vi "Write.vi"(8 "error in (no error)":errorcluster, 10 "Command To Write":string, 11 "VISA resource name":refnum<visa-resource-name>) -> (0 "error out":errorcluster, 3 "VISA resource name out":refnum<visa-resource-name>)   [LabVIEW 2018, in "EFD Ultimus V.lvlib"]
doc: "Writes a command to the Ultimus V unit, computes the checksum and sets the command to the correct format. For example, acceptable inputs are EK-- , UCccc, E8ccc. Refer to the Ultimus V manual for host format command formats."
uses:
  EFD Ultimus V.lvlib
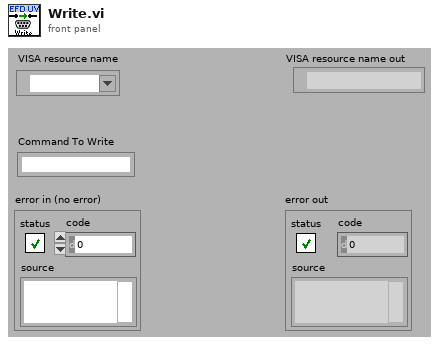
[diagram p1: front panel]
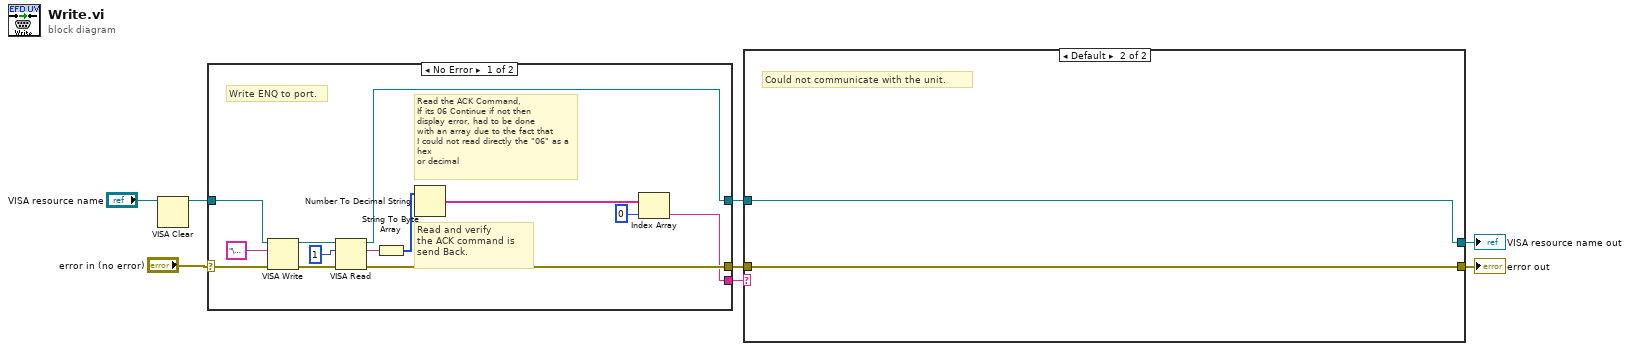
[diagram p0: block diagram]
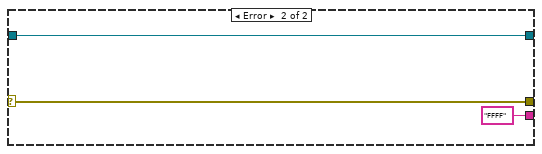
[diagram p2: hidden frame]
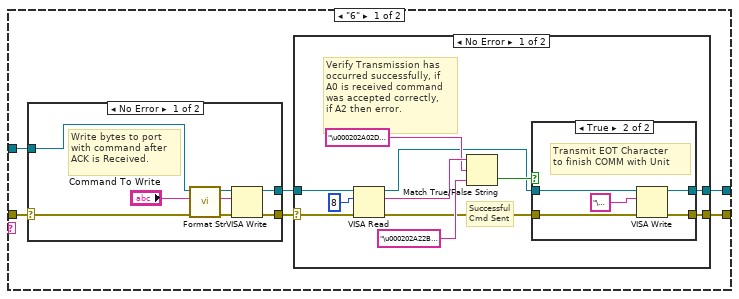
[diagram p3: hidden frame]
diagram:
  n1 = VISA Clear(VISA resource name="VISA resource name") -> (VISA resource name out=w4:refnum<visa-resource-name>)  [unwired: 1 in, 1 out]
  n2 = case shown="No Error" "error in (no error)" {
    selector: "error in (no error)" -> [w21 w24]
    tunnel: [w15 w23] -> w5
    tunnel: [w16 w24] -> w6
    tunnel: w4 -> [w20 w23]
    tunnel: [w10 "FFFF" ("read buffer")] -> w7
    frame No Error {
      # "Read the ACK Command,\nIf its 06 Continue if not then\ndisplay error, had to be done\nwith an array due to the fact that \nI could not read directly the \"06\" as a hex\nor decimal"
      # "Read and verify \nthe ACK command is \nsend Back."
      # "Write ENQ to port."
      n3 = VISA Write(VISA resource name=w20, write buffer="\u0005", error in (no error)=w21) -> (VISA resource name out=w18:refnum<visa-resource-name>, error out=w17:errorcluster)  [unwired: 1 out]
      n4 = VISA Read(VISA resource name=w18, byte count=u32 1, error in (no error)=w17) -> (VISA resource name out=w15:refnum<visa-resource-name>, read buffer=w14:string, error out=w16:errorcluster)  [unwired: 1 out]
      n5 = String To Byte Array(string=w14) -> (unsigned byte array=w13:u8[])
      n6 = Number To Decimal String(number=w13) -> (decimal integer string=w12:string[])  [unwired: 1 out]
      n7 = Index Array(array=w12, index=0) -> (element=w10:string)
    }
    frame Error {
    }
  }
  n8 = case shown="Default" w7 {
    tunnel: [w26 w62] -> w8
    tunnel: w5 -> [w28 w62]
    tunnel: w6 -> [w27 w61]
    tunnel: [w25 w61] -> w1
    frame "6" {
      n9 = case shown="No Error" w27 {
        selector: w27 -> [w56 w60]
        tunnel: [w57 w59] -> w30
        tunnel: [w58 w60] -> w29
        tunnel: w28 -> [w52 w59]
        frame No Error {
          # "Write bytes to port\nwith command after\nACK is Received."
          n10 = call "Format Str.vi"("error in (no error)"=w56, "Input Cmd String"="Command To Write", "VISA resource name"=w52) -> ("error out"=w55:errorcluster, "Formatted Cmd String"=w54:string, "VISA resource name out"=w51:refnum<visa-resource-name>)  [unwired: 6 in]
          n11 = VISA Write(VISA resource name=w51, write buffer=w54, error in (no error)=w55) -> (VISA resource name out=w57:refnum<visa-resource-name>, error out=w58:errorcluster)  [unwired: 1 out]
        }
        frame Error {
        }
      }
      n12 = case "Read bytes from port." shown="No Error" w29 {
        selector: w29 -> [w40 w49]
        tunnel: [w31 w49] -> w25
        tunnel: [w33 w50] -> w26
        tunnel: w30 -> [w41 w50]
        frame No Error {
          # "Verify Transmission has\noccurred successfully, if\nA0 is received command\nwas accepted correctly,\nif A2 then error."
          # "Successful \nCmd Sent"
          n13 = VISA Read(VISA resource name=w41, byte count=u32 8, error in (no error)=w40) -> (VISA resource name out=w34:refnum<visa-resource-name>, read buffer=w39:string, error out=w32:errorcluster)  [unwired: 1 out]
          n14 = Match True/False String(2:"\u000202A22B\u0003" ("false string"), 3:"\u000202A02D\u0003" ("true string"), 4:w39) -> (0:w35:bool)  [unwired: 1 out]
          n15 = case shown="True" w35 {
            tunnel: w34 -> [w43 w47]
            tunnel: [w43 w48] -> w33
            tunnel: w32 -> [w42 w46]
            tunnel: [w42 w45] -> w31
            frame False {
            }
            frame True {
              # "Transmit EOT Character\nto finish COMM with Unit"
              n16 = VISA Write(VISA resource name=w47, write buffer="\u0004", error in (no error)=w46) -> (VISA resource name out=w48:refnum<visa-resource-name>, error out=w45:errorcluster)  [unwired: 1 out]
            }
          }
        }
        frame Error {
          # "Error occurred \nreading Bytes at \nSerial Port"
        }
      }
    }
    frame Default {
      # "Could not communicate with the unit."
    }
  }
  "VISA resource name out" <- w8
  "error out" <- w1
